vi "5.7.5-Midbrain-Act-UDPServer.vi"() -> ()   [LabVIEW 2010]
doc: "Creates a named service and listens on the first available port. Whenever a client connects to the service, it responds with a message containing joystick data. The VI can be stopped using the STOP button."
uses:
  4-High Neurons/4.1-Act Control Typedef.ctl
  4-High Neurons/4.1.0-Datatype Typedef.ctl
  5.0-Global.vi
panel:
  out "5.6.4 Act Control":T1
  out "data out":string
  out "error out":errorcluster
  in  "error in":errorcluster
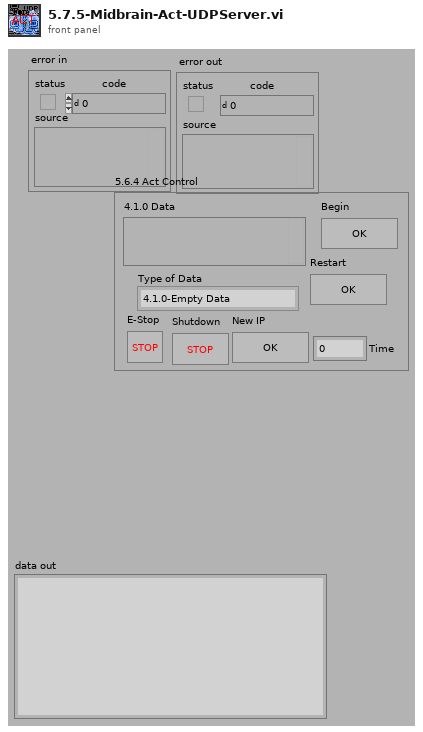
[diagram p1: front panel]
types:
  T1 = typedef "4.1-Act Control Typedef.ctl" = cluster{"4.1.0 Data":variant, "Type of Data":T2, "E-Stop":bool, "Restart":bool, "New IP":bool, "Begin":bool, "Time":i32, "Shutdown":bool}
  T2 = typedef "4.1.0-Datatype Typedef.ctl" = enum16{"4.1.0-Empty Data", "4.1.1-Joystick Data", "4.1.2-Behavioral Data"}
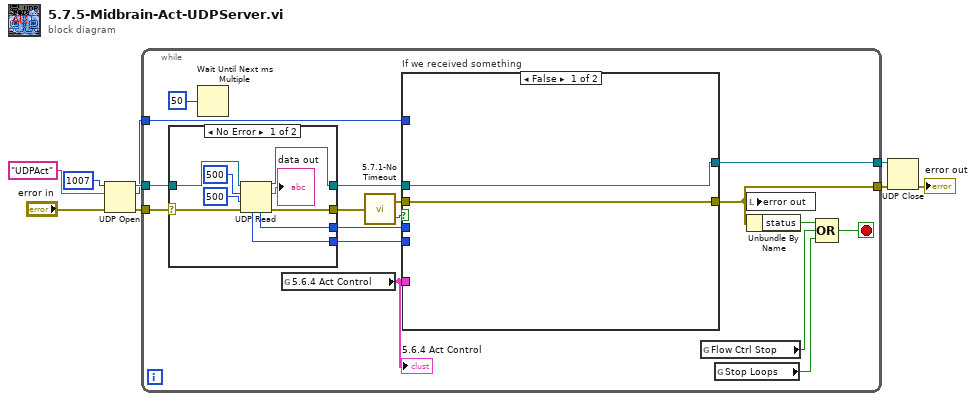
[diagram p0: block diagram]
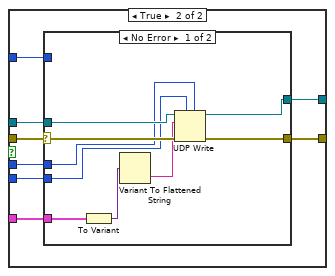
[diagram p2: hidden frame]
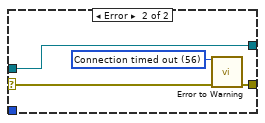
[diagram p3: hidden frame]
diagram:
  n1 = UDP Open(8:"error in", 10:"UDPAct", 11:u16 1007 ("port")) -> (port=w8:refnum<k16>, 0:w7:errorcluster, 2:w3:u16)  [unwired: 2 in]
  n2 = while {
    tunnel: [w15] -> w5
    tunnel: w8 -> [w26]
    tunnel: w7 -> [w23]
    tunnel: [w24] -> w6
    tunnel: w3 -> [w20]
    stop <- w18 stop-if-true
    n3 = case shown="No Error" w23 {
      selector: w23 -> [w56 w59]
      tunnel: w26 -> [w58 w60]
      tunnel: [w55 w60] -> w25
      tunnel: [w54 w59] -> w14
      tunnel: [w52 _] -> w21
      tunnel: [w53 _] -> w22
      frame No Error {
        n4 = UDP Read(connection ID=w58, max size (548)=500, timeout ms (25000)=500, 8:w56) -> (data out=→"data out":string, error out=w54:errorcluster, 3:w55:refnum<k16>, 4:w52:u16, 6:w53:u32)
      }
      frame Error {
      }
    }
    n5 = Wait Until Next ms Multiple(millisecond multiple=u32 50) -> ()  [unwired: 1 out]
    n6 = global read "5.0-Global.vi" "5.6.4 Act Control"() -> (w13:T1)
    "5.6.4 Act Control" <- w13
    n7 = call "5.7.1-No Timeout.vi"("error in (no error)"=w14) -> ("No Timeout"=w16:bool, "error out"=w17:errorcluster)
    n8 = case "If we received something" shown="False" w16 {
      tunnel: w25 -> [w27 w36]
      tunnel: [w27 w35] -> w24
      tunnel: w22 -> [_ w34]
      tunnel: w21 -> [_ w33]
      tunnel: w20 -> [_ w32]
      tunnel: [w28 w31] -> w15
      tunnel: w17 -> [w28 w30]
      tunnel: w13 -> [_ w29]
      frame False {
      }
      frame True {
        n9 = case shown="No Error" w30 {
          selector: w30 -> [w45 w47]
          tunnel: w36 -> [w42 w49]
          tunnel: [w44 w46] -> w31
          tunnel: [w43 w49] -> w35
          tunnel: w34 -> [w40 _]
          tunnel: w33 -> [w41 _]
          tunnel: w32 -> [_ _]
          tunnel: w29 -> [w37 _]
          frame No Error {
            n10 = To Variant(anything=w37) -> (Variant=w39:variant)
            n11 = Variant To Flattened String(Variant=w39) -> (data string=w38:string)  [unwired: 1 out]
            n12 = UDP Write(address=w40, port or service name=w41, connection ID=w42, data in=w38, 8:w45) -> (error out=w44:errorcluster, 3:w43:refnum<k16>)  [unwired: 1 in]
          }
          frame Error {
            w48 = 56 items=["No Error", "Argument Error", "Memory Full", "Out of Zone", "End of File", "File Already Open", "Generic File IO Error", "File Not Found", "File Permission Error", "Disk Full", "Duplicate Path", "Too Many Files Open", "Not Enabled", "Resource File Not Found", "Cannot Add Resource", "Resource Not Found", "Image Not Found", "Image Memory Error", "Pen Does Not Exist", "Config Bad Type", "Config Token Not Found", "Config Parse Error", "Config Memory Error", "Bad External Code Format", "Bad External Code Offset", "External Code Not Present", "Null Window", "Destroy Window Mixup", "Null Menu", "Print Aborted", "Bad Print Record", "Print Driver Error", "Windows Error During Print", "Memory Error During Print", "Print Dialog Error", "Generic Print Error", "Invalid Device Refnum", "Device Not Found", "Device Parameter Error", "Device Unit Error", "Can't Open Device", "Device Call Aborted", "Generic Error", "Cancelled By User", "Object ID Too Low", "Object ID Too High", "Object Not In Heap", "Unknown Heap", "Bad DefProc ID", "DefProc Not In Table", "Message Out Of Range", "Null Method", "Unknown Message", "Manager Call Not Supported", "Bad address", "Connection In progress", "Connection timed out", "Connection is already in progress", "Network attribute not supported", "Network error", "Address in use", "System out of memory", "Connection aborted", "Connection refused", "Connection is not connected", "Connection is already connected", "Connection closed", "Initialize error (interapplication manager)", "Bad occurrence", "Wait on unbound occurrence handler", "Occurrence queue overflow", "Bad path", "Semaphore not signaled", "Unrecognized type (interapplication manager)"] ("1st Error to Convert")
            n13 = call <vilib>:"Error to Warning.vi"("1st Error to Convert"=w48, "error in"=w47) -> ("warning out"=w46:errorcluster)  [unwired: 13 in]
          }
        }
      }
    }
    n14 = global read "5.0-Global.vi" "Flow Ctrl Stop"() -> (w11:bool)
    n15 = global read "5.0-Global.vi" "Stop Loops"() -> (w10:bool)
    n16 = local write "error out"(w15) -> ()
    n17 = Unbundle By Name(w15) -> ("status"=w19:bool)
    n18 = Compound Arithmetic op=OR(w19, w11, w10) -> (w18:bool)
  }
  n19 = UDP Close(connection ID=w6, 8:w5) -> (error out=→"error out":errorcluster)  [unwired: 1 out]
